vi "Session UnLoad.vi"(8 "error in (no error)":errorcluster, 11 "ONNX Class in":refnum<class "ONNX Class.lvclass">) -> (0 "error out":errorcluster, 3 "ONNX Class out":refnum<class "ONNX Class.lvclass">)   [LabVIEW 2017, in "ONNX Class Library.lvlib" / "ONNX Class.lvclass"]
uses:
  ONNX Class.lvclass
  ONNX Class.lvclass/ONNX Class.ctl
  ONNX Class Library.lvlib
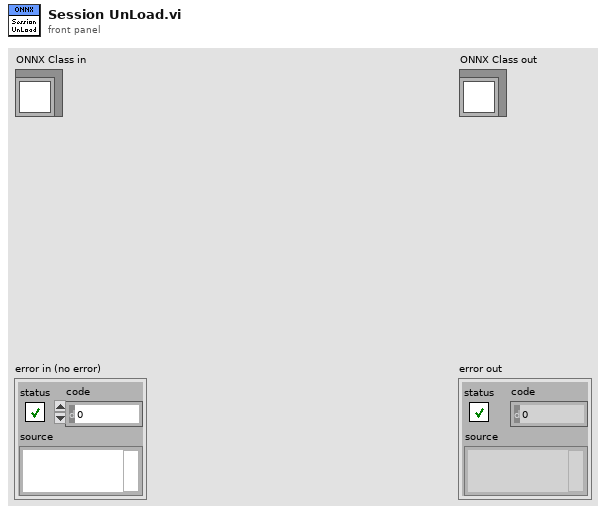
[diagram p1: front panel]
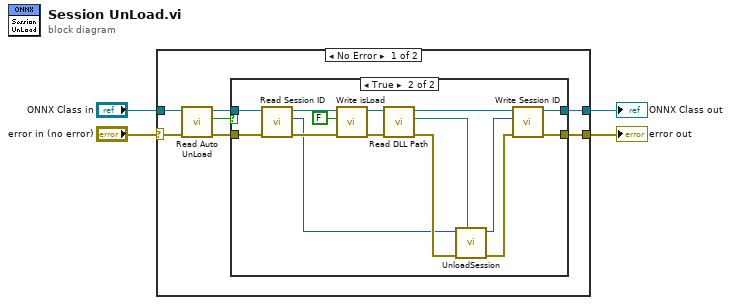
[diagram p0: block diagram]
diagram:
  n1 = case shown="No Error" "error in (no error)" {
    selector: "error in (no error)" -> [w5 w30]
    tunnel: [w7 w30] -> w2
    tunnel: [w10 w29] -> w3
    tunnel: "ONNX Class in" -> [w6 w29]
    frame No Error {
      n2 = call-dynamic "Read Auto UnLoad.vi"("error in (no error)"=w5, "ONNX Class in"=w6) -> ("error out"=w8:errorcluster, "Auto UnLoad"=w9:bool, "ONNX Class out"=w11:refnum<class "ONNX Class.lvclass">)  [unwired: 7 in]
      n3 = case shown="True" w9 {
        tunnel: [w12 w22] -> w7
        tunnel: w11 -> [w13 w27]
        tunnel: [w13 w23] -> w10
        tunnel: w8 -> [w12 w25]
        frame False {
        }
        frame True {
          n4 = call-dynamic "Read Session ID.vi"("error in (no error)"=w25, "ONNX Class in"=w27) -> ("error out"=w24:errorcluster, "Session ID"=w15:i32, "ONNX Class out"=w26:refnum<class "ONNX Class.lvclass">)  [unwired: 7 in]
          n5 = call-dynamic "Write isLoad.vi"("error in (no error)"=w24, "isLoad"=FALSE, "ONNX Class in"=w26) -> ("error out"=w18:errorcluster, "ONNX Class out"=w19:refnum<class "ONNX Class.lvclass">)  [unwired: 7 in]
          n6 = call-dynamic "Read DLL Path.vi"("error in (no error)"=w18, "ONNX Class in"=w19) -> ("error out"=w17:errorcluster, "DLL Path"=w14:path, "ONNX Class out"=w16:refnum<class "ONNX Class.lvclass">)  [unwired: 7 in]
          n7 = call "UnloadSession.vi"("DLL Path"=w14, "error in (no error)"=w17, "session id in"=w15) -> ("error out"=w21:errorcluster, "session id out"=w20:i32)  [unwired: 7 in]
          n8 = call-dynamic "Write Session ID.vi"("error in (no error)"=w21, "Session ID"=w20, "ONNX Class in"=w16) -> ("error out"=w22:errorcluster, "ONNX Class out"=w23:refnum<class "ONNX Class.lvclass">)  [unwired: 7 in]
        }
      }
    }
    frame Error {
    }
  }
  "error out" <- w2
  "ONNX Class out" <- w3
